vi "Measure - NI 9219.vi"(8 "Error In":errorcluster) -> (0 "Error Out":errorcluster)   [LabVIEW 2011]
doc: "This VI will do some basic temperature/voltage measurement with NI 9219."
uses:
  <vilib>/DAQmx/read.llb/DAQmx Read.vi
  <vilib>/DAQmx/read.llb/DAQmx Read (Analog 1D Wfm NChan NSamp).vi
  <vilib>/DAQmx/miscellaneous.llb/DAQmx Fill In Error Info.vi
panel:
  out "Thermometer":dbl(slide) scale=0.0..50.0
  out "data":waveform(dbl)[](graph) caption="Chart"
  in  "stop":bool
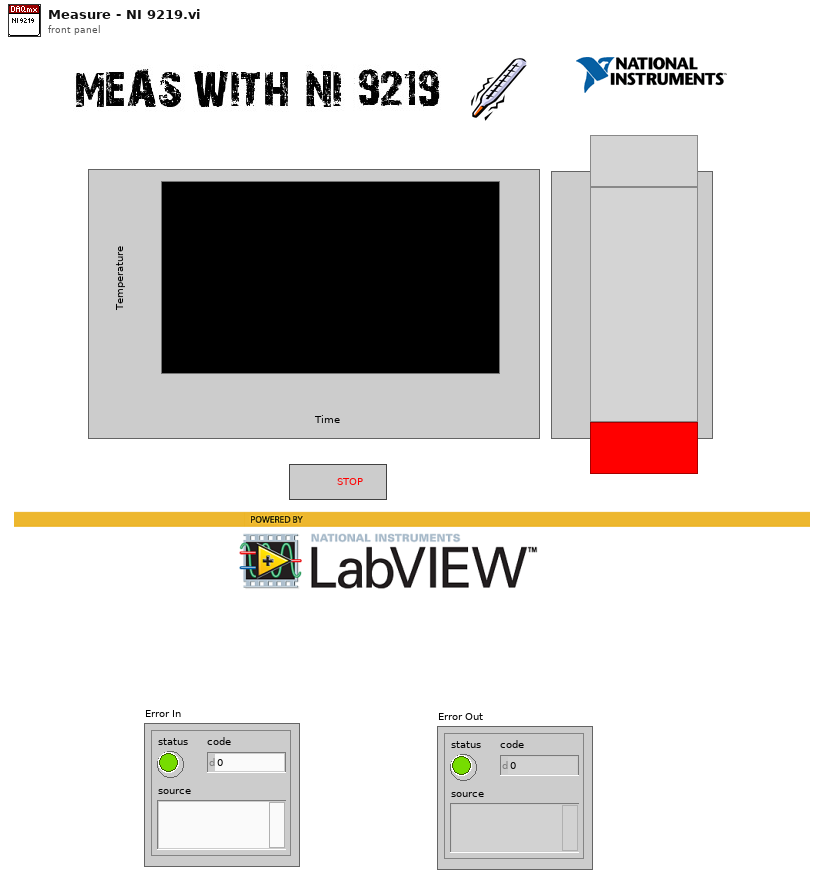
[diagram p1: front panel]
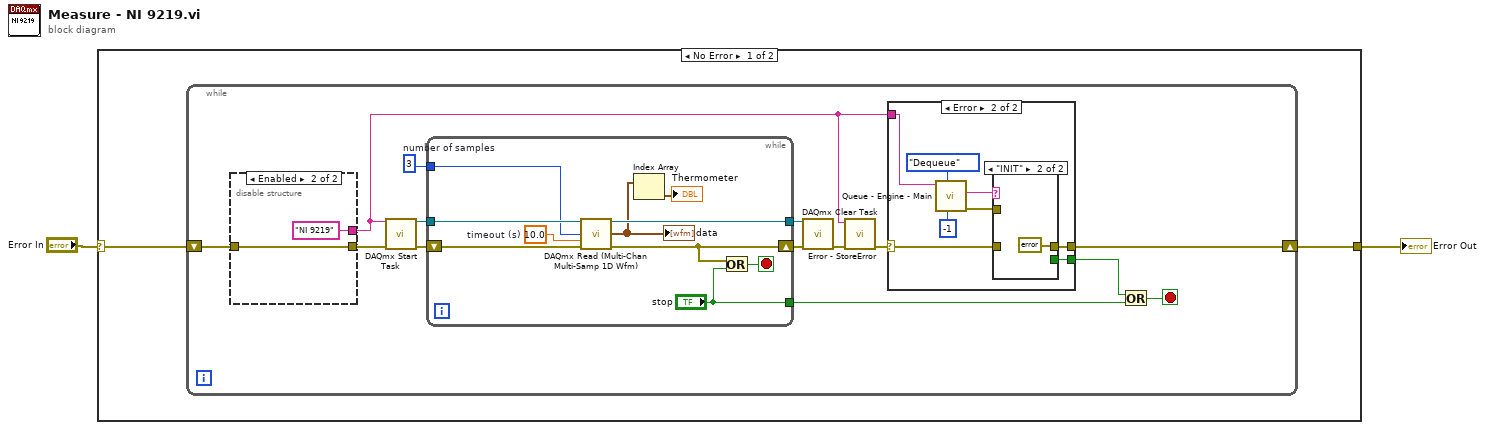
[diagram p0: block diagram]
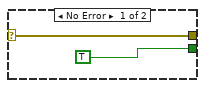
[diagram p2: hidden frame]
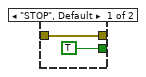
[diagram p3: hidden frame]
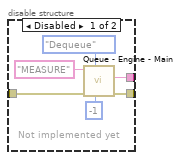
[diagram p4: hidden frame]
diagram:
  n1 = case shown="No Error" "Error In" {
    selector: "Error In" -> [w4 w50]
    tunnel: [w3 w50] -> w2
    frame No Error {
      n2 = while {
        shift-right: [w10] -> w3
        shift-left: w4 -> [w18]
        stop <- w9 stop-if-true
        w15 = 3  # number of samples
        n3 = disable-structure shown="Enabled" {
          disable-tunnel: [w47 w49] -> w12
          disable-tunnel: [w46 "NI 9219" ("Variable In")] -> w5
          disable-tunnel: w18 -> [w45 w49]
          frame Disabled {
            # "Not implemented yet"
            n4 = call "Queue - Engine - Main.vi"("timeout in ms (-1)"=-1, "Operation"=enum16{"Enqueue", "Dequeue", "Flush", "Release"}."Dequeue", "error in"=w45, "Queue Name In"="MEASURE") -> ("error out"=w47:errorcluster, "Data Out"=w46:string)  [unwired: 5 in, 1 out]
          }
          frame Enabled {
          }
        }
        n5 = call <vilib>:"DAQmx Start Task.vi"("task/channels in"=w5, "error in"=w12) -> ("task out"=w17:refnum<k21>, "error out"=w16:errorcluster)  [unwired: 12 out]
        n6 = while {
          tunnel: w17 -> [w40]
          tunnel: w15 -> [w39]
          tunnel: [w36] -> w13
          shift-right: [w37] -> w14
          shift-left: w16 -> [w38]
          tunnel: ["stop"] -> w8
          stop <- w41 stop-if-true
          w35 = 10.0  # timeout (s)
          n7 = call-poly "DAQmx Read (Multi-Chan Multi-Samp 1D Wfm).vi"("task/channels in"=w40, "number of samples per channel"=w39, "timeout"=w35, "error in"=w38) -> ("task out"=w36:refnum<k21>, "data"=w34:waveform(dbl)[], "error out"=w37:errorcluster)  [unwired: 9 out]
          "data" <- w34
          n8 = Index Array(array=w34) -> (element=→"Thermometer":waveform(dbl))  [unwired: 1 in]
          n9 = Or(x=w37, y="stop") -> (x .or. y?=w41:bool)
        }
        n10 = call <vilib>:"DAQmx Clear Task.vi"("task in"=w13, "error in"=w14) -> ("error out"=w11:errorcluster)  [unwired: 13 out]
        n11 = call "Error - StoreError.vi"("Error In"=w11, "Error Source In"=w5) -> ("Error Out"=w7:errorcluster)  [unwired: 8 in, 1 out]
        n12 = case shown="Error" w7 {
          selector: w7 -> [w20 w21]
          tunnel: [w20 w23] -> w10
          tunnel: [TRUE w22] -> w6
          tunnel: w5 -> [_ w26]
          frame No Error {
          }
          frame Error {
            n13 = call "Queue - Engine - Main.vi"("timeout in ms (-1)"=-1, "Operation"=enum16{"Enqueue", "Dequeue", "Flush", "Release"}."Dequeue", "Queue Name In"=w26) -> ("error out"=w25:errorcluster, "Data Out"=w24:string)  [unwired: 6 in, 1 out]
            n14 = case shown="\"INIT\"" w24 {
              tunnel: w25 -> [_ _]
              tunnel: [w29 errorcluster {"status"=FALSE, "code"=0, "source"=""} ("error out")] -> w23
              tunnel: [TRUE _] -> w22
              tunnel: w21 -> [w29 _]
              frame "STOP", Default {
              }
              frame "INIT" {
              }
            }
          }
        }
        n15 = Or(x=w6, y=w8) -> (x .or. y?=w9:bool)
      }
    }
    frame Error {
    }
  }
  "Error Out" <- w2
